vi "get all streams.vi"(8 "error in (no error)":errorcluster, 11 "CD in":T1 format="%.0x") -> (0 "error out":errorcluster, 3 "streams":T1[](array[typedef]) format="%.0x")   [LabVIEW 2026, in "Nominal Core Streaming Shared.lvlib"]
uses:
  Nominal Core Streaming Shared.lvlib
  <vilib>/NI VeriStand/Custom Device Tools/Custom Device Utility Library/Custom Device Utility Library.lvlib
  <vilib>/NI VeriStand/Custom Device Tools/Custom Device Utility Library/NI VeriStand - Search for All Items by GUID.vi
  Constants.vi
  <vilib>/NI VeriStand/Custom Device API/Custom Device Item Ref.ctl
  <vilib>/NI VeriStand/Custom Device API/Custom Device API.lvlib
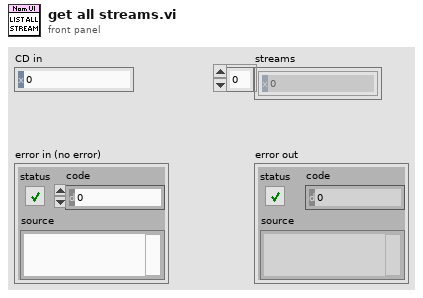
[diagram p1: front panel]
types:
  T1 = typedef "Custom Device API.lvlib/Custom Device Item Ref.ctl" = u64
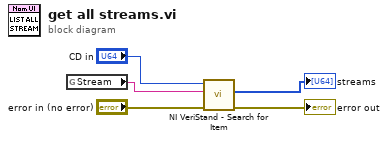
[diagram p0: block diagram]
diagram:
  n1 = global read "Constants.vi" "Stream"() -> (w1:string)
  n2 = call-poly <vilib>:"NI VeriStand - Search for Item.vi"("error in"="error in (no error)", "Item GUID"=w1, "Section Ref in"="CD in") -> ("error out"=→"error out":errorcluster, "Item Refs"=→"streams":T1[])  [unwired: 5 in, 2 out]
